vi "Log sweep.vi"(1 "Stop frequency":dbl, 2 "Start frequency":dbl, 3 "Number of points":i32=2 min=2) -> (0 "log10 space out":dbl[](array[numeric]))   [LabVIEW 2017]
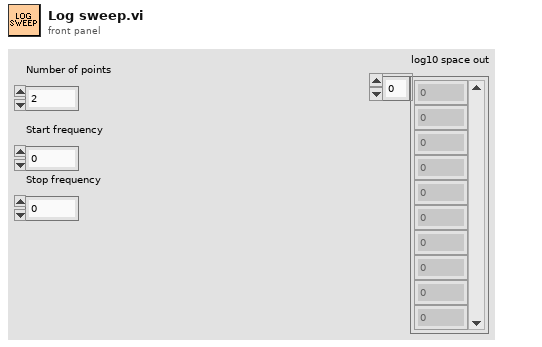
[diagram p1: front panel]
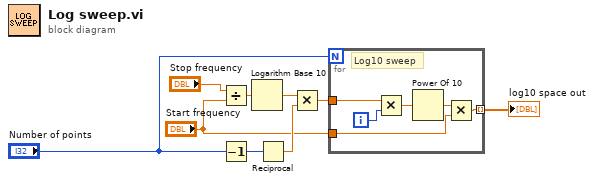
[diagram p0: block diagram]
diagram:
  n1 = Divide(x="Stop frequency", y="Start frequency") -> (x/y=w3:dbl)
  n2 = Decrement(x="Number of points") -> (x-1=w8:i32)
  n3 = Logarithm Base 10(1:w3) -> (0:w4:dbl)
  n4 = Reciprocal(x=w8) -> (1/x=w6:dbl)
  n5 = Multiply(x=w4, y=w6) -> (x*y=w5:dbl)
  n6 = for {
    N: "Number of points" -> [_]
    tunnel: w5 -> [w14]
    tunnel: [w11] -> w7 mode=indexing
    tunnel: "Start frequency" -> [w10]
    i -> [w15]
    # "Log10 sweep"
    n7 = Multiply(x=w14, y=w15) -> (x*y=w13:dbl)
    n8 = Power Of 10(x=w13) -> (10^x=w12:dbl)
    n9 = Multiply(x=w12, y=w10) -> (x*y=w11:dbl)
  }
  "log10 space out" <- w7
